vi "SDO download (U8).vi"(6 "Value":u8, 7 "Wait?":bool, 8 "error in (no error)":errorcluster, 9 "Multiplexor":T1 {"Index" format="%04x"}, 10 "Node ID":u8, 11 "CANopen in":refnum<class "CANopen.lvclass">) -> (0 "error out":errorcluster, 3 "CANopen out":refnum<class "CANopen.lvclass">)   [LabVIEW 2024, in "canopen.lvlib" / "CANopen.lvclass"]
doc: "Writes a value in the open dictionary of a CANopen node."
uses:
  CANopen.lvclass
  CANopen.lvclass/CANopen.ctl
  Multiplexor.ctl
  CANopen Master.lvlib
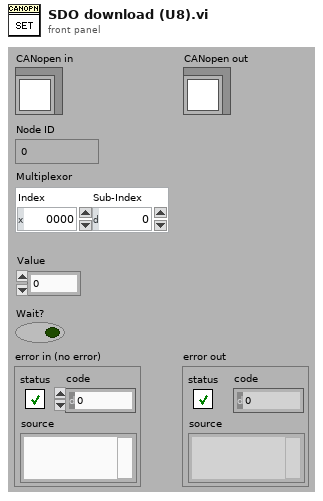
[diagram p1: front panel]
types:
  T1 = typedef "CANopen Master.lvlib/Multiplexor.ctl" = cluster{"Index":u16, "Sub-Index":u8}
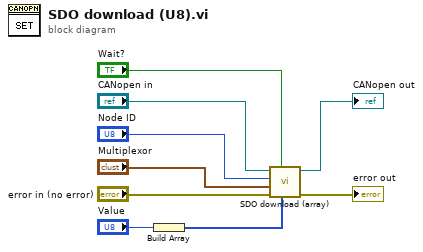
[diagram p0: block diagram]
diagram:
  n1 = Build Array("Value") -> (w2:u8[])
  n2 = call "SDO download (array).vi"("Value"=w2, "Wait?"="Wait?", "error in (no error)"="error in (no error)", "Multiplexor"="Multiplexor", "Node ID"="Node ID", "CANopen in"="CANopen in") -> ("error out"=→"error out":errorcluster, "CANopen out"=→"CANopen out":refnum<class "CANopen.lvclass">)  [unwired: 2 out]
